vi "Test Loess Smoothing.vi"() -> ()   [LabVIEW 2015]
uses:
  LinSpace (x0-dx-npts).vi
  <vilib>/Analysis/NI_AALBase.lvlib
panel:
  in  "Robust?":bool
  in  "Quadratic?":bool
  in  "Span":i32
  out "Waveform Graph":dbl[][](graph)
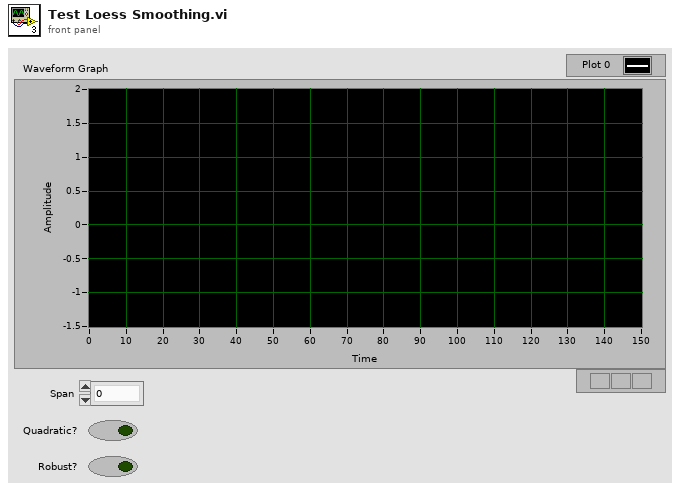
[diagram p1: front panel]
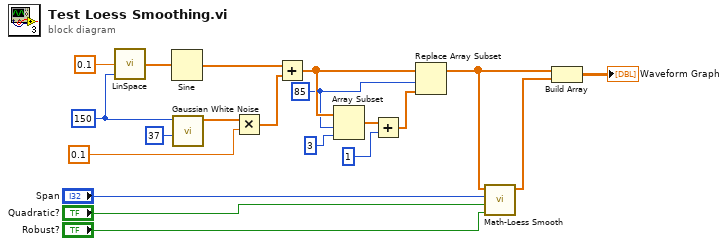
[diagram p0: block diagram]
diagram:
  w1 = 85 ("index")
  w18 = 150 ("npts")
  n1 = call-poly "LinSpace.vi"("npts"=w18, "dx"=0.1) -> ("Array"=w19:dbl[])  [unwired: 2 in, 1 out]
  n2 = Sine(x=w19) -> (sin(x)=w15:dbl[])
  n3 = call <vilib>:"Gaussian White Noise.vi"("seed"=37, "samples"=w18) -> ("Gaussian noise pattern"=w17:dbl[])  [unwired: 8 in, 1 out]
  n4 = Multiply(x=w17, y=0.1) -> (x*y=w14:dbl[])
  n5 = Add(x=w15, y=w14) -> (x+y=w4:dbl[])
  n6 = Array Subset(array=w4, index=w1, length=3) -> (w6:dbl[])
  n7 = Add(x=w6, y=1) -> (x+y=w2:dbl[])
  n8 = Replace Array Subset(array=w4, new element=w2, index=w1) -> (w3:dbl[])
  n9 = call "Math-Loess Smooth.vi"("Robust?"="Robust?", "Quadratic?"="Quadratic?", "Span"="Span", "Array"=w3) -> ("Smoothed Array"=w12:dbl[])  [unwired: 7 in]
  n10 = Build Array(w3, w12) -> (→"Waveform Graph":dbl[][])
